vi "_poll_scan.vi"(8 "error in (no error)":errorcluster, 11 "UV-VIS_AVANTES in":refnum<class "UV-VIS_AVANTES.lvclass">) -> (0 "error out":errorcluster, 2 "return":i32, 3 "UV-VIS_AVANTES out":refnum<class "UV-VIS_AVANTES.lvclass">)   [LabVIEW 2020, in "UV-VIS_AVANTES.lvclass"]
uses:
  UV-VIS_AVANTES.lvclass
  C:/dev/TRANCON/Classes/Detector/Detector.lvclass
  Detector.lvclass/Detector.ctl
  UV-VIS_AVANTES.lvclass/UV-VIS_AVANTES.ctl
  Detector.lvclass
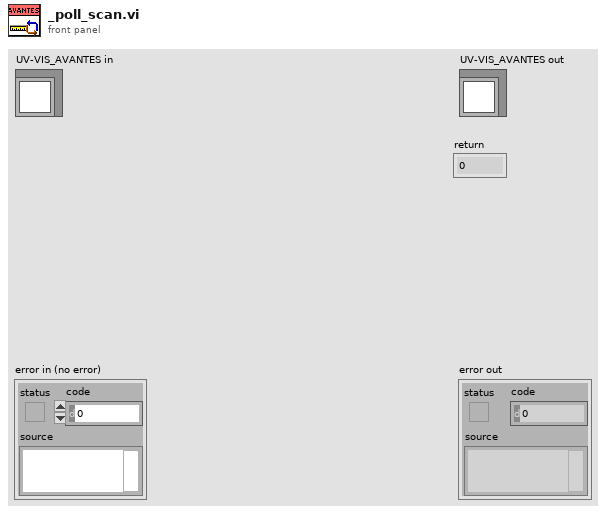
[diagram p1: front panel]
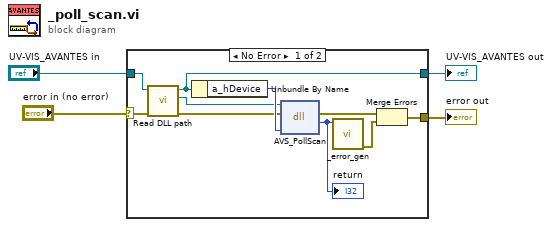
[diagram p0: block diagram]
diagram:
  n1 = case shown="No Error" "error in (no error)" {
    selector: "error in (no error)" -> [w13 w16]
    tunnel: [w11 w16] -> w3
    tunnel: [w12 w15] -> w1
    tunnel: "UV-VIS_AVANTES in" -> [w14 w15]
    frame No Error {
      n2 = call "Read DLL path.vi"("error in (no error)"=w13, "Detector in"=w14) -> ("error out"=w9:errorcluster, "DLL path"=w8:path, "Detector out"=w12:refnum<class "UV-VIS_AVANTES.lvclass">)  [unwired: 7 in]
      n3 = Unbundle By Name(w12) -> ("a_hDevice"=w10:i32)
      n4 = dll-call lib="C:/AvaSpecX64-DLL_9.4/examples/LabView/LabViewSingleChan/avaspec.dll" fn="AVS_PollScan"(path in=w8, error in=w9, "a_hDevice"=w10) -> (error out=w5:errorcluster, "return type"=w7:i32)  [unwired: 2 in, 1 out]
      "return" <- w7
      n5 = call "_error_gen.vi"("return type"=w7) -> ("error out"=w6:errorcluster)  [unwired: 10 in]
      n6 = Merge Errors(w5, w6) -> (w11:errorcluster)
    }
    frame Error {
    }
  }
  "error out" <- w3
  "UV-VIS_AVANTES out" <- w1
